vi "Encode GND Parameters.vi"(6 "scanner? (F:No)":bool, 8 "ADD Parameters in":string, 9 "Scanner Selection in (0)":i32, 11 "GND Test Parameters in":T1={"Current (25 A)"=25.0, "Voltage (8 V)"=8.0, "Hi-Limit (100 mohm)"=100.0, "Lo-Limit (0 mohm)"=0.0, "Dwell (1 s)"=1.0, "Offset (0 mohm)"=0.0, "Auto Offset (OFF)"=FALSE} {"Offset (0 mohm)" format="%#.2f"; "Lo-Limit (0 mohm)" format="%#.2f"; "Hi-Limit (100 mohm)" format="%#.2f"}) -> (0 "Scanner Selection out":i32, 1 "GND Test Parameters Out":T1={"Current (25 A)"=25.0, "Voltage (8 V)"=8.0, "Hi-Limit (100 mohm)"=100.0, "Lo-Limit (0 mohm)"=0.0, "Dwell (1 s)"=1.0, "Offset (0 mohm)"=0.0, "Auto Offset (OFF)"=FALSE} {"Offset (0 mohm)" format="%#.2f"; "Lo-Limit (0 mohm)" format="%#.2f"; "Hi-Limit (100 mohm)" format="%#.2f"}, 3 "ADD Parameters out":string)   [LabVIEW 2014]
doc: "GND Test Parameters in: Converts test parameters to ADD2 string used to ADD/Edit steps.\n\nADD Parameters in: Decodes LS2? responces to test parameters."
uses:
  <instrlib>/EEC EST 300/Public/Configure/Steps/Low Level/GND Test Parameters.ctl
  <instrlib>/eec EST 300/eec EST 300.lvlib
panel:
  # "ON"
  # "OFF"
  # "ON"
  # "OFF"
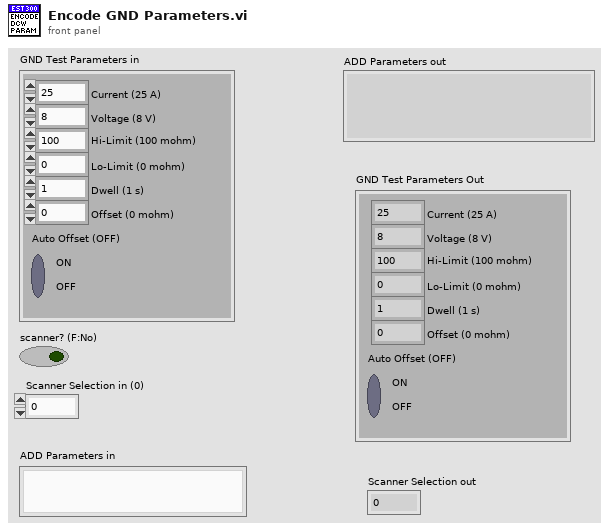
[diagram p1: front panel]
types:
  T1 = typedef "EEC EST 300.lvlib/GND Test Parameters.ctl" = cluster{"Current (25 A)":dbl, "Voltage (8 V)":dbl, "Hi-Limit (100 mohm)":dbl, "Lo-Limit (0 mohm)":dbl, "Dwell (1 s)":dbl, "Offset (0 mohm)":dbl, "Auto Offset (OFF)":bool}
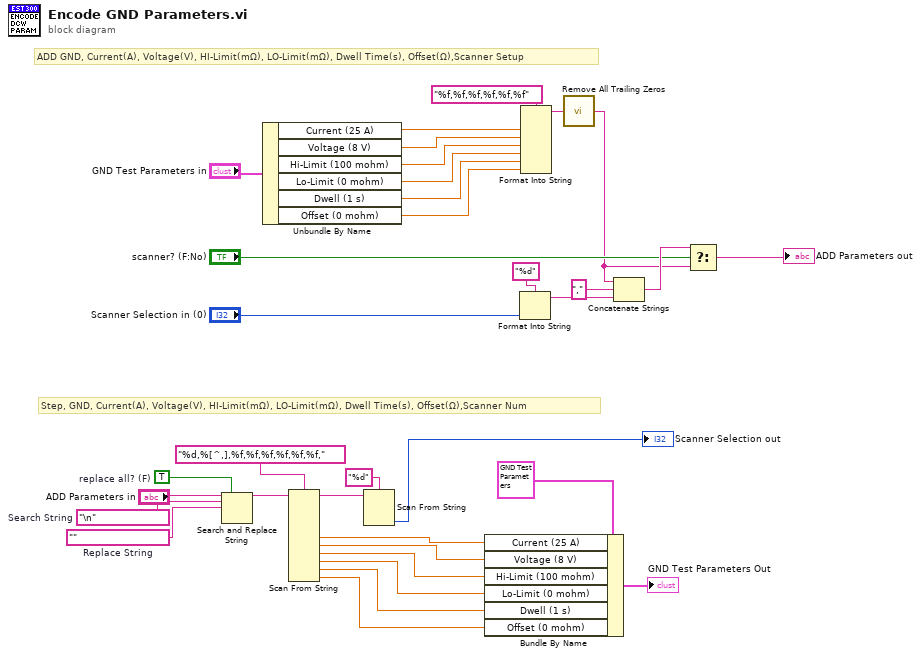
[diagram p0: block diagram]
diagram:
  w26 = TRUE  # replace all? (F)
  w20 = ""  # Replace String
  w27 = "\n"  # Search String
  # "Step, GND, Current(A), Voltage(V), HI-Limit(mΩ), LO-Limit(mΩ), Dwell Time(s), Offset(Ω),Scanner Num"
  # "ADD GND, Current(A), Voltage(V), HI-Limit(mΩ), LO-Limit(mΩ), Dwell Time(s), Offset(Ω),Scanner Setup"
  n1 = Search and Replace String(replace all?=w26, input string="ADD Parameters in", search string=w27, replace string=w20) -> (result string=w25:string)  [unwired: 4 in, 3 out]
  n2 = Unbundle By Name("GND Test Parameters in") -> ("Current (25 A)"=w28:dbl, "Voltage (8 V)"=w21:dbl, "Hi-Limit (100 mohm)"=w22:dbl, "Lo-Limit (0 mohm)"=w34:dbl, "Dwell (1 s)"=w33:dbl, "Offset (0 mohm)"=w32:dbl)
  n3 = Scan From String(format string="%d,%[^,],%f,%f,%f,%f,%f,%f," ("Format String"), input string=w25) -> (remaining string=w7:string, output 3=w13:dbl, output 4=w12:dbl, output 5=w11:dbl, output 6=w10:dbl, output 7=w9:dbl, output 8=w8:dbl)  [unwired: 12 in, 2 out]
  n4 = Scan From String(format string="%d", input string=w7) -> (output 1=→"Scanner Selection out":i32)  [unwired: 3 in, 3 out]
  n5 = Bundle By Name(cluster=T1 {"Current (25 A)"=25.0, "Voltage (8 V)"=8.0, "Hi-Limit (100 mohm)"=100.0, "Lo-Limit (0 mohm)"=0.0, "Dwell (1 s)"=1.0, "Offset (0 mohm)"=0.0, "Auto Offset (OFF)"=FALSE} ("GND Test Parameters Out"), "Current (25 A)"=w13, "Voltage (8 V)"=w12, "Hi-Limit (100 mohm)"=w11, "Lo-Limit (0 mohm)"=w10, "Dwell (1 s)"=w9, "Offset (0 mohm)"=w8) -> (→"GND Test Parameters Out":T1)
  n6 = Format Into String(format string="%d", "Scanner Selection in (0)") -> (resulting string=w16:string)  [unwired: 2 in, 1 out]
  n7 = Format Into String(format string="%f,%f,%f,%f,%f,%f" ("Format String"), w28, w21, w22, w34, w33, w32) -> (resulting string=w2:string)  [unwired: 2 in, 1 out]
  n8 = call <instrlib>:"Remove All Trailing Zeros.vi"("String in"=w2) -> ("String out"=w1:string)
  n9 = Concatenate Strings(w1, "," ("Substring"), w16) -> (w24:string)
  n10 = Select(t=w24, s="scanner? (F:No)", f=w1) -> (s? t:f=→"ADD Parameters out":string)
